vi "JL_Obtain Dryness LED Config.vi"(0 "Dryness Option":u8 format="%x") -> (4 "Fail":bool, 6 "Pass":bool, 8 "Dryness LED Config":T1=enum."Damp")   [LabVIEW 2016]
uses:
  type defs/Dryness Enum.ctl
panel:
  # "All integers are hex"
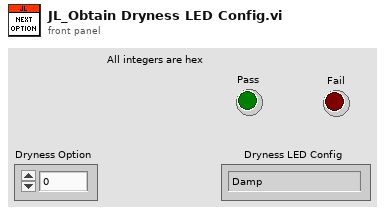
[diagram p1: front panel]
types:
  T1 = typedef "Dryness Enum.ctl" = enum16{"Off", "Damp", "Less Dry", "Dry", "More Dry", "Extra Dry", "*Incorrect*"}
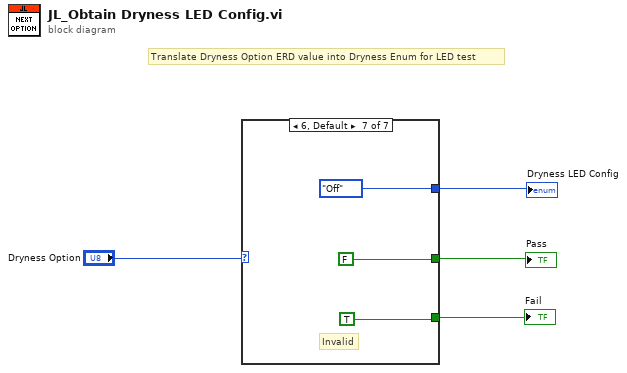
[diagram p0: block diagram]
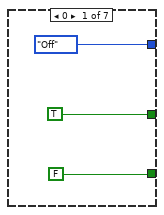
[diagram p2: hidden frame]
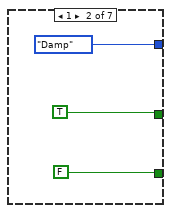
[diagram p3: hidden frame]
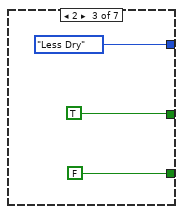
[diagram p4: hidden frame]
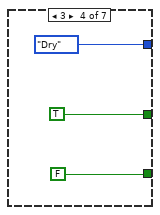
[diagram p5: hidden frame]
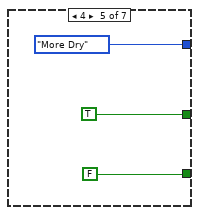
[diagram p6: hidden frame]
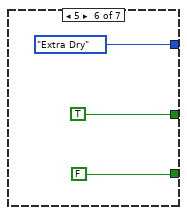
[diagram p7: hidden frame]
diagram:
  # "Translate Dryness Option ERD value into Dryness Enum for LED test"
  n1 = case shown="6, Default" "Dryness Option" {
    tunnel: [Dryness_Enum."Off" ("Dryness Level 2") Dryness_Enum."Damp" ("Dryness Level 2") Dryness_Enum."Less Dry" ("Dryness Level 2") Dryness_Enum."Dry" ("Dryness Level 2") Dryness_Enum."More Dry" ("Dryness Level 2") Dryness_Enum."Extra Dry" ("Dryness Level 2") Dryness_Enum."Off" ("Dryness Level 2")] -> w4
    tunnel: [TRUE ("Pass 2") TRUE ("Pass 2") TRUE ("Pass 2") TRUE ("Pass 2") TRUE ("Pass 2") TRUE ("Pass 2") FALSE ("Pass 2")] -> w2
    tunnel: [FALSE ("Pass 2") FALSE ("Pass 2") FALSE ("Pass 2") FALSE ("Pass 2") FALSE ("Pass 2") FALSE ("Pass 2") TRUE ("Pass 2")] -> w1
    frame 0 {
    }
    frame 1 {
    }
    frame 2 {
    }
    frame 3 {
    }
    frame 4 {
    }
    frame 5 {
    }
    frame 6, Default {
      # "Invalid"
    }
  }
  "Dryness LED Config" <- w4
  "Pass" <- w2
  "Fail" <- w1
